vi "driveSimple.vi"(10 "Speed (ft/sec)":dbl, 11 "Distance":dbl) -> ()   [LabVIEW 2011]
uses:
  drivetrain/gear_shift_state.ctl
  drivetrain/drivetrain_drive_mode.ctl
  drivetrain/drivetrain_drive_write_thread.ctl
  drivetrain/drivetrain_globals.vi
panel:
  in  "time_slow":u32=400
  in  "speed_cal":dbl=2.5
  in  "time_start_cal":u32=600
  out "Distance (in)":cluster{"Left":dbl, "Right":dbl}
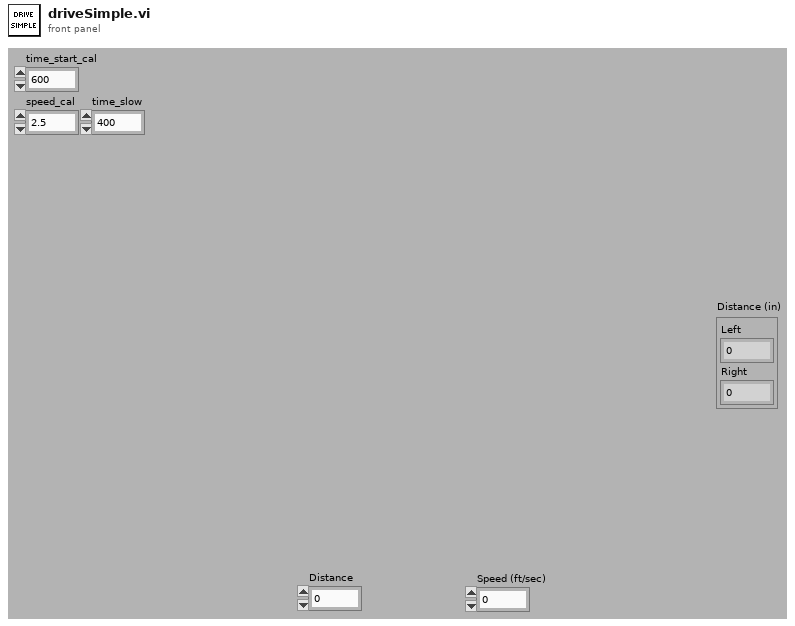
[diagram p1: front panel]
types:
  T1 = typedef "gear_shift_state.ctl" = enum16{"low", "high"}
  T2 = typedef "drivetrain_drive_mode.ctl" = enum16{"open loop", "closed loop"}
  T3 = typedef "drivetrain_drive_write_thread.ctl" = enum16{"Teleop", "Script Engine - Autonomous", "Script Engine - Sequence"}
  T4 = typedef "WPI_RobotDriveDevRef.ctl" = cluster{"DevStatus":errorcluster, "Motors[]":T5[], "Square Inputs":bool, "Max Output":dbl}
  T5 = typedef "WPI_MotorControlDeviceRef.ctl" = cluster{"DeviceStatus":errorcluster, "Type":enum16{"PWM", "CAN"}, "PWM":cluster{"Digital Module":T6, "PWM Channel":T7, "DeadBand":T8}, "CAN":cluster{"Device Number":u8, "Control Mode":T9, "Semaphore":T10, "Max Vout":dbl}, "Invert":bool, "TransformRef":T11, "InvTransformRef":T11}
  T6 = typedef "FPGA_TypedefDigitalModule.ctl" = enum16{"Digital Module 1", "Digital Module 2"}
  T7 = typedef "FPGA_DIOPWMChannel.ctl" = enum8{"PWM 1", "PWM 2", "PWM 3", "PWM 4", "PWM 5", "PWM 6", "PWM 7", "PWM 8", "PWM 9", "PWM 10", "Invalid"}
  T8 = typedef "WPI_PWMDeadband.ctl" = cluster{"Name":string, "maxPositivePwm":i32, "minPositivePwm":i32, "centerPwm":i32, "maxNegativePwm":i32, "minNegativePwm":i32, "angularRange":u16}
  T9 = typedef "WPI_CANJaguar_ControlMode.ctl" = enum8{"Percent VBus", "Current", "Speed", "Position", "Voltage"}
  T10 = typedef "Semaphore RefNum" = refnum<k1>
  T11 = typedef "WPI_PWMTransform_ConPane.ctl" = refnum<vi>
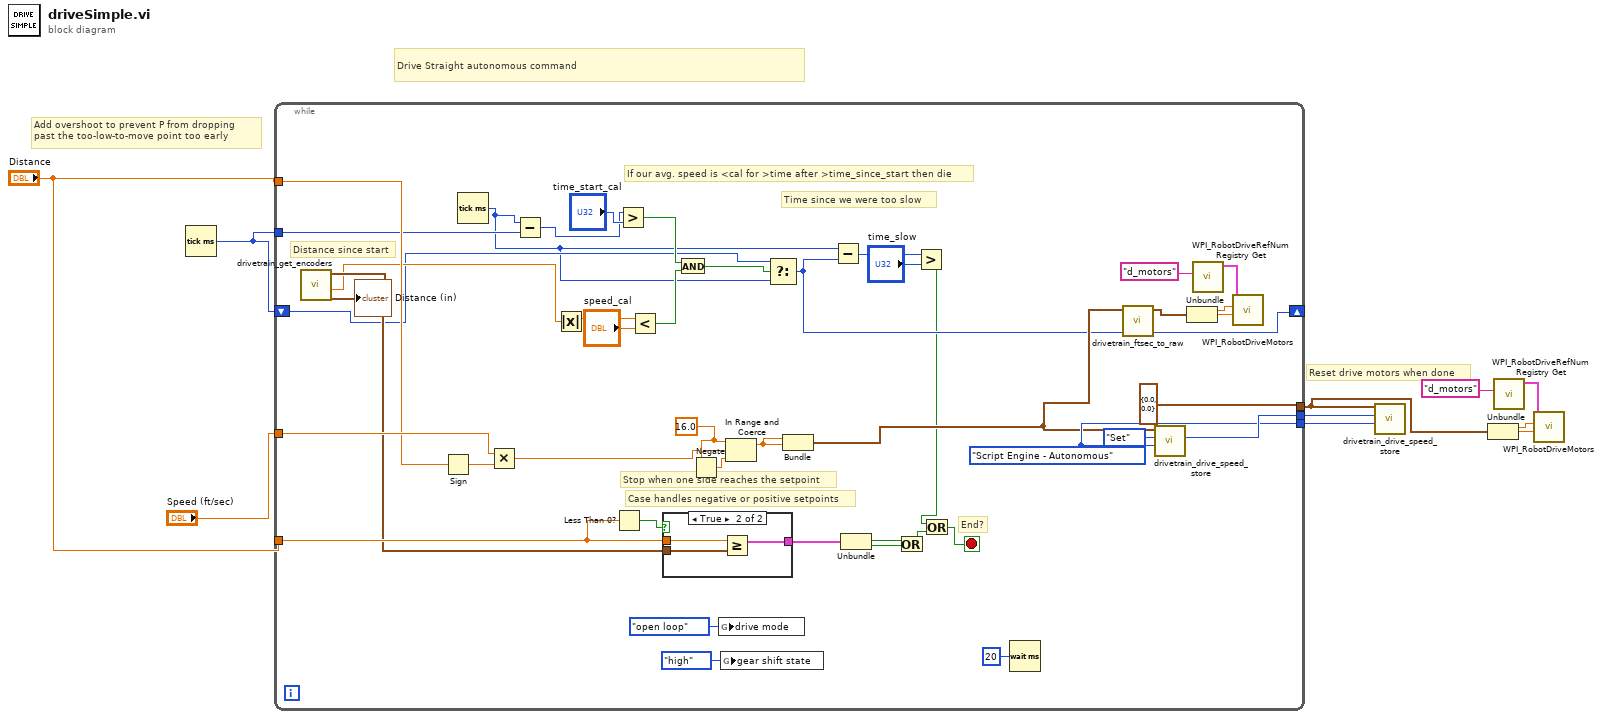
[diagram p0: block diagram]
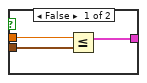
[diagram p2: hidden frame]
diagram:
  # "Drive Straight autonomous command"
  # "Reset drive motors when done"
  # "Add overshoot to prevent P from dropping\npast the too-low-to-move point too early"
  n1 = Tick Count (ms)() -> (millisecond timer value=w1:u32)
  n2 = while {
    tunnel: "Speed (ft/sec)" -> [w42]
    tunnel: "Distance" -> [w40]
    tunnel: [cluster{"Left":dbl, "Right":dbl} {"Left"=0.0, "Right"=0.0} ("Drive")] -> w5
    tunnel: "Distance" -> [w44]
    tunnel: [w38] -> w9
    tunnel: [w37] -> w8
    tunnel: w1 -> [w27]
    shift-right: [w13] -> _
    shift-left: w1 -> [w19]
    stop <- w14 stop-if-true
    w37 = drivetrain_drive_write_thread."Script Engine - Autonomous" ("Write Thread")
    w38 = enum16{"Set", "Get"}."Set" ("data_store_mode")
    w45 = 16.0
    # "Time since we were too slow"
    # "If our avg. speed is <cal for >time after >time_since_start then die"
    # "Case handles negative or positive setpoints"
    # "End?"
    # "Stop when one side reaches the setpoint"
    # "Distance since start"
    n3 = call "drivetrain_get_encoders.vi"() -> ("Avg Velocity (Ft/Sec)"=w26:dbl, "Distance (in)"=w35:cluster{"Left":dbl, "Right":dbl})  [unwired: 9 in, 1 out]
    "Distance (in)" <- w35
    n4 = Sign(1:w40) -> (0:w39:dbl)
    n5 = Tick Count (ms)() -> (millisecond timer value=w11:u32)
    n6 = Multiply(x=w42, y=w39) -> (x*y=w41:dbl)
    n7 = Subtract(x=w11, y=w27) -> (x-y=w18:u32)
    n8 = Absolute Value(x=w26) -> (abs(x)=w25:dbl)
    n9 = Less Than 0?(x=w44) -> (x < 0?=w47:bool)
    n10 = Greater?(x=w18, y="time_start_cal") -> (0:w22:bool)
    n11 = Less?(x=w25, y="speed_cal") -> (x < y?=w21:bool)
    n12 = case shown="True" w47 {
      tunnel: w44 -> [w55 w58]
      tunnel: w35 -> [w54 w57]
      tunnel: [w53 w56] -> w52
      frame False {
        n13 = Less Or Equal?(x=w55, y=w54) -> (x <= y?=w53:cluster{"Left":bool, "Right":bool})
      }
      frame True {
        n14 = Greater Or Equal?(x=w58, y=w57) -> (x >= y?=w56:cluster{"Left":bool, "Right":bool})
      }
    }
    n15 = And(x=w22, y=w21) -> (x .and. y?=w20:bool)
    n16 = Negate(x=w45) -> (-x=w46:dbl)
    n17 = global write "drivetrain_globals.vi" "drive mode"(drivetrain_drive_mode."open loop" ("drive mode")) -> ()
    n18 = global write "drivetrain_globals.vi" "gear shift state"(gear_shift_state."high" ("gear shift state")) -> ()
    n19 = In Range and Coerce(upper limit=w45, x=w41, lower limit=w46) -> (coerced(x)=w43:dbl)  [unwired: 1 out]
    n20 = Select(t=w19, s=w20, f=w11) -> (s? t:f=w13:u32)
    n21 = Bundle(w43, w43) -> (w28:cluster{dbl, dbl})  [unwired: 1 out]
    n22 = Subtract(x=w11, y=w13) -> (x-y=w17:u32)
    n23 = Unbundle(w52) -> ("Left"=w51:bool, "Right"=w50:bool)
    n24 = Or(x=w51, y=w50) -> (x .or. y?=w15:bool)
    n25 = Greater?(x=w17, y="time_slow") -> (0:w12:bool)
    n26 = Or(x=w12, y=w15) -> (x .or. y?=w14:bool)
    n27 = Wait (ms)(milliseconds to wait=u32 20) -> ()  [unwired: 1 out]
    n28 = call "drivetrain_ftsec_to_raw.vi"("Drive Data"=w28) -> ("Drive Data Out"=w29:cluster{"Left":dbl, "Right":dbl})  [unwired: 10 in]
    n29 = call "drivetrain_drive_speed_store.vi"("Write Thread"=w37, "data_store_mode"=w38, "drive data"=w28) -> ()  [unwired: 7 in, 2 out]
    n30 = Unbundle(w29) -> ("Left"=w31:dbl, "Right"=w32:dbl)
    n31 = call <vilib>:"WPI_RobotDriveRefNum Registry Get.vi"("refnum name"="d_motors") -> ("RobotDriveDevRef"=w34:T4)  [unwired: 9 in, 1 out]
    n32 = call <vilib>:"WPI_RobotDriveMotors.vi"("RightSpeed"=w32, "LeftSpeed"=w31, "RobotDriveDevRef"=w34) -> ()  [unwired: 7 in, 2 out]
  }
  n33 = call "drivetrain_drive_speed_store.vi"("Write Thread"=w8, "data_store_mode"=w9, "drive data"=w5) -> ()  [unwired: 7 in, 2 out]
  n34 = Unbundle(w5) -> ("Left"=w7:dbl, "Right"=w6:dbl)
  n35 = call <vilib>:"WPI_RobotDriveRefNum Registry Get.vi"("refnum name"="d_motors") -> ("RobotDriveDevRef"=w3:T4)  [unwired: 9 in, 1 out]
  n36 = call <vilib>:"WPI_RobotDriveMotors.vi"("RightSpeed"=w6, "LeftSpeed"=w7, "RobotDriveDevRef"=w3) -> ()  [unwired: 7 in, 2 out]
